vi "Main_22b.vi"() -> ()   [LabVIEW 2023]
uses:
  Cluster_Node.ctl
panel:
  out "Brick Map":map{i32, T1[]}(c390)
  out "Grid":i32[][][](array[numeric])
  out "Array 2":i32[][](array[numeric])
  out "Answer":i32
  in  "Puzzle":string="5,5,156~5,7,156\n8,5,82~8,7,82\n6,5,196~6,7,196\n0,7,7~0,8,7\n2,3,129~2,6,129\n9,5,265~9,7,265\n1,4,278~3,4,278\n2,6,149~4,6,149\n7,7,246~9,7,246\n8,6,282~9,6,282\n1,1,289~1,5,289\n7,3,70~7,6,70\n3,9,278~3,9,280\n6,9,261~7,9,261\n3,5,75~5,5,75\n3,1,221~3,1,224\n0,9,211~2,9,211\n3,9,251~4,9,251\n0,4,28~2,4,28\n2,7,291~2,7,293\n4,3,2~4,5,2\n5,4,96~5,5,96\n5,4,60~5,7,60\n1,2,45~4,2,45\n3,6,145~3,9,145\n9,1,214~9,4,214\n0,4,121~0,6,121\n6,5,22~8,5,22\n2,8,211~4,8,211\n5,0,215~6,0,215\n7,1,80~7,4,80\n4,9,2~6,9,2\n5,8,13~7,8,13\n0,9,210~3,9,210\n6,6,107~6,8,107\n6,7,228~6,9,228\n0,9,96~2,9,96\n0,0,101~0,0,102\n6,4,108~6,6,108\n5,2,237~5,2,240\n1,5,200~1,8,200\n5,9,210~8,9,210\n2,0,28~2,2,28\n2,5,222~4,5,222\n6,7,59~8,7,59\n9,8,152~9,9,152\n0,1,205~0,3,205\n8,7,49~9,7,49\n4,1,44~4,1,47\n0,5,65~0,7,65\n2,2,303~2,3,303\n6,6,21~6,9,21\n4,4,99~4,7,99\n1,0,155~4,0,155\n7,5,15~9,5,15\n4,5,232~4,7,232\n1,9,213~1,9,215\n1,3,105~1,5,105\n4,6,197~4,7,197\n0,6,235~0,7,235\n8,4,303~8,6,303\n3,7,62~5,7,62\n4,2,279~7,2,279\n4,0,45~6,0,45\n8,7,195~8,9,195\n1,7,88~5,7,88\n1,0,246~4,0,246\n5,6,115~5,6,118\n3,3,25~3,5,25\n1,7,261~4,7,261\n7,3,206~8,3,206\n4,1,49~6,1,49\n7,1,179~9,1,179\n6,1,264~8,1,264\n1,8,205~4,8,205\n4,5,283~5,5,283\n3,3,208~3,5,208\n4,1,101~4,1,102\n2,2,272~2,2,274\n4,7,43~4,9,43\n5,7,188~5,9,188\n6,8,290~6,9,290\n3,6,111~6,6,111\n3,4,230~5,4,230\n5,7,154~7,7,154\n8,5,83~9,5,83\n4,2,283~6,2,283\n7,3,276~7,6,276\n6,0,270~8,0,270\n7,7,77~9,7,77\n2,0,256~2,0,258\n3,3,305~3,5,305\n9,7,87~9,9,87\n1,9,219~1,9,221\n3,3,123~3,6,123\n2,2,194~2,2,195\n7,5,64~7,5,67\n1,8,89~1,9,89\n1,0,291~1,2,291\n0,9,166~1,9,166\n2,6,274~2,9,274\n0,6,17~0,6,20\n5,6,277~8,6,277\n4,2,227~4,4,227\n4,6,8~4,7,8\n5,4,84~7,4,84\n1,6,266~1,9,266\n0,7,228~2,7,228\n8,5,29~8,8,29\n1,9,230~2,9,230\n2,1,140~2,3,140\n1,6,3~3,6,3\n2,8,3~2,9,3\n4,0,161~4,2,161\n2,6,254~3,6,254\n5,0,32~5,2,32\n4,0,205~4,2,205\n0,1,161~1,1,161\n2,0,21~5,0,21\n3,1,132~5,1,132\n9,1,10~9,1,10\n7,2,89~7,4,89\n6,0,170~9,0,170\n8,0,145~8,3,145\n1,1,5~3,1,5\n3,5,13~3,7,13\n3,1,30~7,1,30\n7,6,175~7,6,178\n8,4,3~8,5,3\n5,3,113~7,3,113\n2,5,120~3,5,120\n0,0,20~0,3,20\n5,7,47~8,7,47\n3,5,171~3,5,173\n5,4,128~5,7,128\n8,9,211~9,9,211\n3,1,297~5,1,297\n1,9,102~3,9,102\n4,2,47~4,2,47\n4,6,302~4,9,302\n9,3,88~9,3,90\n5,0,26~5,3,26\n7,1,84~8,1,84\n8,1,263~8,3,263\n8,0,95~9,0,95\n2,4,116~2,6,116\n6,4,171~8,4,171\n7,4,245~7,7,245\n4,1,33~6,1,33\n2,2,147~2,4,147\n0,2,276~3,2,276\n5,2,266~8,2,266\n1,3,274~3,3,274\n3,6,193~3,6,196\n0,2,35~3,2,35\n5,4,311~5,5,311\n6,2,274~6,5,274\n9,0,126~9,2,126\n3,4,112~3,6,112\n5,5,163~8,5,163\n6,0,88~8,0,88\n4,0,214~7,0,214\n5,2,35~7,2,35\n4,8,66~7,8,66\n0,8,165~1,8,165\n0,6,180~2,6,180\n4,0,104~6,0,104\n0,5,270~0,8,270\n4,2,73~4,4,73\n3,2,17~5,2,17\n1,5,168~3,5,168\n7,7,22~8,7,22\n6,3,2~6,5,2\n8,3,123~8,5,123\n6,9,142~6,9,143\n7,1,310~9,1,310\n7,1,203~7,4,203\n5,3,272~5,7,272\n1,3,22~1,3,22\n0,9,153~3,9,153\n2,3,285~4,3,285\n1,0,56~1,3,56\n1,8,105~1,9,105\n8,1,128~9,1,128\n1,0,13~1,0,16\n0,6,153~0,8,153\n2,5,95~2,7,95\n6,8,265~8,8,265\n2,1,200~5,1,200\n4,2,307~4,2,309\n1,0,243~3,0,243\n7,1,307~7,4,307\n3,5,99~3,5,102\n3,0,106~4,0,106\n0,1,321~3,1,321\n2,3,199~2,4,199\n6,0,283~6,1,283\n7,2,38~9,2,38\n8,5,16~9,5,16\n0,2,37~0,3,37\n2,2,312~4,2,312\n6,1,225~6,3,225\n1,9,263~1,9,265\n1,6,87~1,8,87\n4,6,40~4,8,40\n4,9,45~7,9,45\n3,1,177~3,1,178\n8,7,14~9,7,14\n4,8,214~7,8,214\n4,7,224~4,9,224\n1,2,245~1,3,245\n8,3,260~8,6,260\n7,7,278~7,8,278\n3,6,212~7,6,212\n0,2,18~0,3,18\n4,6,122~6,6,122\n2,5,12~2,6,12\n7,6,275~7,9,275\n5,5,249~8,5,249\n6,2,83~9,2,83\n4,2,316~6,2,316\n2,6,15~2,6,15\n6,6,248~7,6,248\n7,3,280~9,3,280\n4,8,275~6,8,275\n0,0,77~0,2,77\n6,5,63~8,5,63\n5,0,37~5,0,40\n6,1,75~6,4,75\n4,0,38~4,0,40\n0,8,99~3,8,99\n4,1,298~6,1,298\n7,8,268~9,8,268\n9,1,313~9,3,313\n4,8,24~6,8,24\n5,6,264~5,9,264\n8,3,32~8,5,32\n2,0,205~2,0,207\n0,2,8~2,2,8\n2,7,102~2,7,104\n1,8,239~2,8,239\n8,6,201~9,6,201\n2,1,202~3,1,202\n3,9,62~5,9,62\n8,5,8~8,5,10\n3,9,158~4,9,158\n9,2,143~9,4,143\n8,4,81~8,6,81\n3,9,2~3,9,2\n4,4,67~6,4,67\n3,4,199~3,7,199\n6,8,274~9,8,274\n6,5,58~8,5,58\n9,3,28~9,6,28\n3,1,104~4,1,104\n8,6,23~8,7,23\n2,9,136~4,9,136\n7,0,167~7,3,167\n5,3,11~7,3,11\n6,2,76~6,2,79\n9,0,216~9,2,216\n3,2,255~3,3,255\n0,3,127~0,4,127\n0,1,209~3,1,209\n5,7,191~5,8,191\n5,3,134~5,6,134\n9,2,150~9,2,152\n2,1,295~4,1,295\n1,6,56~1,7,56\n1,9,93~5,9,93\n1,3,24~4,3,24\n5,1,133~7,1,133\n6,8,175~9,8,175\n0,8,272~0,8,274\n0,7,14~0,9,14\n1,7,297~4,7,297\n8,5,68~8,8,68\n2,0,247~5,0,247\n7,2,3~7,2,6\n0,7,247~0,9,247\n4,0,288~6,0,288\n4,6,71~7,6,71\n4,1,57~4,1,59\n2,1,92~4,1,92\n0,4,41~0,6,41\n3,8,287~5,8,287\n3,6,184~5,6,184\n4,3,54~4,4,54\n0,1,208~4,1,208\n0,2,46~1,2,46\n8,4,69~8,5,69\n5,6,113~5,8,113\n6,3,260~6,4,260\n7,3,83~7,4,83\n4,1,170~7,1,170\n0,1,224~0,2,224\n0,4,89~0,6,89\n1,0,9~2,0,9\n6,5,278~6,5,281\n5,2,45~8,2,45\n3,8,155~5,8,155\n2,3,20~4,3,20\n9,2,270~9,4,270\n0,2,127~1,2,127\n1,6,228~3,6,228\n2,3,30~2,5,30\n1,4,124~1,4,126\n1,0,162~1,1,162\n7,2,69~7,3,69\n5,6,198~7,6,198\n2,3,3~2,5,3\n8,1,269~9,1,269\n8,2,146~8,2,147\n0,0,221~3,0,221\n3,8,176~6,8,176\n3,3,83~3,6,83\n7,0,122~8,0,122\n4,4,164~6,4,164\n6,1,106~6,3,106\n3,8,150~5,8,150\n0,6,303~0,7,303\n3,2,205~3,5,205\n4,1,296~4,4,296\n1,8,245~1,9,245\n9,4,156~9,6,156\n6,2,137~6,2,139\n0,3,125~0,5,125\n0,3,29~2,3,29\n0,5,301~3,5,301\n3,9,275~4,9,275\n6,2,173~6,4,173\n8,4,66~8,7,66\n8,8,26~8,9,26\n5,1,90~6,1,90\n2,6,90~4,6,90\n3,4,75~4,4,75\n0,7,239~2,7,239\n6,1,93~6,4,93\n4,4,100~4,4,101\n1,7,67~3,7,67\n4,5,30~4,7,30\n7,2,31~7,4,31\n6,8,221~6,9,221\n6,2,179~8,2,179\n4,7,218~7,7,218\n9,6,277~9,9,277\n2,3,165~2,7,165\n3,4,131~3,4,131\n0,8,243~3,8,243\n0,6,21~0,9,21\n6,0,2~8,0,2\n3,7,101~3,9,101\n4,2,282~5,2,282\n1,5,203~2,5,203\n5,0,172~8,0,172\n7,3,121~7,5,121\n4,0,95~4,2,95\n3,2,313~4,2,313\n8,3,158~8,3,160\n0,5,36~3,5,36\n2,4,80~2,7,80\n0,6,233~0,8,233\n8,0,71~8,2,71\n8,3,307~8,3,307\n4,1,116~4,3,116\n4,2,21~4,2,23\n0,1,227~0,4,227\n1,7,268~1,8,268\n2,6,10~2,8,10\n8,1,131~8,5,131\n3,2,113~5,2,113\n7,7,280~7,9,280\n1,0,130~1,2,130\n3,8,16~5,8,16\n0,3,82~0,4,82\n9,1,315~9,2,315\n4,3,282~6,3,282\n1,5,10~1,7,10\n8,6,97~8,7,97\n0,0,26~0,1,26\n5,0,46~8,0,46\n5,3,36~5,5,36\n7,1,316~7,3,316\n6,6,172~8,6,172\n6,4,56~6,7,56\n2,0,29~3,0,29\n6,1,15~6,3,15\n6,7,102~6,9,102\n0,4,10~2,4,10\n8,2,216~8,3,216\n4,3,70~4,6,70\n0,9,92~1,9,92\n7,1,79~9,1,79\n0,4,285~0,6,285\n2,2,27~2,4,27\n0,2,83~0,4,83\n7,7,228~7,9,228\n9,4,309~9,4,311\n2,0,107~2,1,107\n2,3,293~2,5,293\n7,4,116~8,4,116\n7,4,166~8,4,166\n6,3,78~9,3,78\n3,4,239~5,4,239\n3,2,212~3,4,212\n0,6,147~2,6,147\n0,2,155~0,5,155\n9,4,314~9,7,314\n5,8,137~5,8,138\n8,5,98~8,8,98\n7,7,178~7,8,178\n1,0,58~1,4,58\n7,1,172~7,4,172\n9,6,252~9,6,254\n6,2,287~8,2,287\n0,0,62~2,0,62\n1,5,59~1,7,59\n1,2,249~1,2,250\n1,7,303~1,9,303\n6,3,138~6,3,140\n6,6,113~6,8,113\n6,0,173~7,0,173\n3,4,189~5,4,189\n5,3,247~8,3,247\n6,3,193~6,3,195\n9,2,75~9,2,76\n6,4,140~8,4,140\n4,1,134~4,1,137\n1,6,297~2,6,297\n4,0,165~6,0,165\n0,2,229~0,4,229\n7,5,150~7,7,150\n0,6,230~0,7,230\n2,3,269~5,3,269\n2,7,49~4,7,49\n0,1,216~2,1,216\n8,0,87~8,2,87\n1,0,157~2,0,157\n4,7,130~4,9,130\n5,2,108~5,3,108\n0,6,130~2,6,130\n0,5,33~3,5,33\n2,6,32~5,6,32\n1,6,89~1,6,91\n4,3,275~4,4,275\n3,6,231~6,6,231\n5,3,301~8,3,301\n2,6,173~4,6,173\n2,8,260~4,8,260\n9,3,199~9,6,199\n0,0,255~2,0,255\n3,3,214~3,3,217\n4,7,249~4,9,249\n2,7,271~4,7,271\n1,2,162~1,4,162\n1,4,117~1,7,117\n0,0,219~0,1,219\n4,6,91~7,6,91\n1,1,85~1,4,85\n8,2,128~9,2,128\n7,7,262~9,7,262\n3,3,8~3,3,10\n2,7,242~3,7,242\n8,4,164~8,6,164\n9,2,87~9,2,87\n2,5,256~4,5,256\n7,0,104~9,0,104\n3,8,60~4,8,60\n7,4,115~9,4,115\n1,0,11~1,2,11\n9,7,142~9,7,145\n3,8,17~3,8,20\n2,4,294~4,4,294\n6,5,220~7,5,220\n2,9,22~2,9,25\n4,0,102~7,0,102\n3,7,22~3,7,24\n5,8,199~7,8,199\n0,6,237~0,6,240\n7,6,17~9,6,17\n1,6,196~1,6,198\n8,0,117~8,3,117\n4,4,33~4,4,35\n7,5,307~7,6,307\n5,6,125~5,9,125\n5,2,216~5,2,217\n0,3,294~0,6,294\n4,8,206~7,8,206\n1,3,102~1,5,102\n3,8,63~4,8,63\n9,4,29~9,4,31\n1,0,248~1,2,248\n0,1,282~0,3,282\n2,7,18~2,9,18\n8,4,307~8,6,307\n1,5,40~2,5,40\n5,4,161~5,6,161\n4,8,134~7,8,134\n8,3,64~8,6,64\n0,7,119~0,8,119\n9,6,255~9,6,257\n3,5,98~3,8,98\n6,3,153~8,3,153\n9,0,25~9,3,25\n2,6,296~2,9,296\n4,9,96~5,9,96\n9,1,283~9,4,283\n9,6,120~9,9,120\n4,7,65~5,7,65\n5,9,293~7,9,293\n6,7,151~7,7,151\n4,7,68~6,7,68\n5,2,190~5,5,190\n8,0,80~8,2,80\n4,4,129~6,4,129\n6,3,303~6,6,303\n9,7,219~9,8,219\n4,1,56~5,1,56\n6,3,290~7,3,290\n6,6,101~6,8,101\n8,3,209~8,4,209\n0,8,170~1,8,170\n6,4,13~7,4,13\n2,1,17~2,3,17\n1,6,189~4,6,189\n6,6,209~6,9,209\n8,3,81~9,3,81\n6,2,107~8,2,107\n2,5,286~5,5,286\n6,7,198~6,9,198\n8,6,199~8,7,199\n1,0,3~1,3,3\n3,1,324~5,1,324\n9,5,197~9,6,197\n3,2,79~5,2,79\n9,7,89~9,9,89\n3,8,282~3,9,282\n1,6,176~3,6,176\n7,0,268~9,0,268\n6,3,134~6,6,134\n0,0,252~1,0,252\n5,3,38~8,3,38\n8,0,183~8,1,183\n0,5,16~0,7,16\n3,0,108~4,0,108\n4,9,64~6,9,64\n2,3,143~4,3,143\n0,7,301~2,7,301\n5,9,13~5,9,15\n2,0,78~5,0,78\n2,2,133~4,2,133\n2,9,228~4,9,228\n5,5,34~5,7,34\n5,7,257~5,9,257\n8,3,30~8,5,30\n3,6,96~5,6,96\n3,5,202~6,5,202\n7,0,218~8,0,218\n8,8,88~8,9,88\n5,4,98~7,4,98\n9,0,5~9,2,5\n4,5,87~4,7,87\n0,2,297~0,4,297\n3,7,64~3,8,64\n1,1,234~2,1,234\n6,3,298~6,3,300\n4,7,285~4,9,285\n4,6,227~6,6,227\n4,5,225~4,6,225\n0,2,249~0,4,249\n5,2,107~5,4,107\n6,2,23~9,2,23\n4,8,145~4,9,145\n5,0,285~7,0,285\n1,4,267~1,6,267\n6,3,97~6,5,97\n9,2,173~9,5,173\n6,3,223~6,5,223\n2,0,240~2,2,240\n1,5,259~3,5,259\n5,5,221~5,8,221\n5,4,124~7,4,124\n0,8,187~2,8,187\n7,2,289~7,3,289\n7,3,10~7,4,10\n6,5,175~6,7,175\n7,2,204~7,4,204\n2,4,155~2,4,157\n4,4,209~4,6,209\n4,1,230~4,3,230\n0,6,246~0,9,246\n0,8,16~0,9,16\n4,4,38~4,4,40\n2,6,138~2,9,138\n7,4,174~7,4,176\n5,6,16~8,6,16\n8,1,110~8,1,112\n9,4,141~9,6,141\n3,5,39~3,5,39\n1,4,9~1,7,9\n0,0,122~0,4,122\n5,2,196~5,4,196\n3,3,54~3,3,56\n1,6,226~3,6,226\n9,1,276~9,3,276\n9,7,15~9,9,15\n2,3,295~2,5,295\n8,4,138~8,7,138\n9,2,281~9,3,281\n4,5,292~4,5,293\n2,4,118~2,6,118\n5,0,111~5,2,111\n9,5,63~9,7,63\n4,1,177~6,1,177\n6,2,25~6,3,25\n5,8,56~7,8,56\n9,9,153~9,9,155\n5,1,213~5,3,213\n1,2,301~2,2,301\n5,1,234~5,3,234\n6,1,204~6,2,204\n7,6,45~7,6,45\n6,5,24~6,7,24\n6,2,259~9,2,259\n1,5,154~1,8,154\n4,0,18~4,2,18\n7,6,174~7,9,174\n2,5,82~4,5,82\n9,6,52~9,9,52\n2,9,156~3,9,156\n5,2,72~7,2,72\n3,6,148~3,8,148\n6,1,114~8,1,114\n0,2,167~0,4,167\n1,1,213~1,3,213\n0,1,10~0,3,10\n7,0,215~9,0,215\n7,5,131~7,7,131\n3,0,9~3,1,9\n2,6,57~2,9,57\n4,3,272~4,5,272\n6,0,52~6,0,54\n4,6,246~4,8,246\n1,9,133~4,9,133\n6,4,77~6,4,77\n1,7,230~2,7,230\n9,4,86~9,5,86\n6,8,78~6,9,78\n2,1,206~5,1,206\n5,8,288~8,8,288\n8,5,125~9,5,125\n0,6,175~0,7,175\n6,3,76~9,3,76\n3,3,104~6,3,104\n3,9,11~5,9,11\n1,6,236~1,8,236\n5,4,246~7,4,246\n1,8,168~3,8,168\n0,5,202~0,7,202\n2,0,200~2,0,201\n9,4,216~9,5,216\n9,8,178~9,8,180\n1,2,280~1,5,280\n6,6,153~9,6,153\n1,2,19~1,4,19\n6,6,219~6,8,219\n5,9,77~7,9,77\n0,7,60~0,8,60\n1,6,199~1,8,199\n0,3,158~2,3,158\n2,4,126~4,4,126\n2,4,225~2,7,225\n8,7,284~9,7,284\n3,6,52~3,8,52\n8,1,182~8,1,182\n2,5,264~2,8,264\n6,5,225~6,5,225\n4,6,41~6,6,41\n0,7,162~3,7,162\n0,4,196~0,6,196\n5,9,83~8,9,83\n3,7,11~5,7,11\n0,7,13~2,7,13\n5,0,160~5,0,162\n1,4,277~3,4,277\n7,1,104~7,1,107\n6,3,269~6,4,269\n5,6,5~5,8,5\n3,9,8~6,9,8\n3,0,1~3,2,1\n1,7,175~3,7,175\n3,3,151~6,3,151\n7,1,158~9,1,158\n6,3,12~7,3,12\n0,1,164~0,2,164\n9,4,175~9,5,175\n3,9,64~3,9,66\n1,8,172~3,8,172\n3,5,41~3,5,41\n8,4,292~8,4,295\n0,6,74~0,8,74\n9,3,83~9,4,83\n4,4,31~4,5,31\n6,0,264~8,0,264\n4,3,21~5,3,21\n3,8,10~5,8,10\n3,9,283~5,9,283\n2,3,304~4,3,304\n0,3,208~0,3,210\n6,4,111~6,4,113\n3,3,75~5,3,75\n3,9,272~5,9,272\n2,6,248~4,6,248\n3,9,265~5,9,265\n9,0,26~9,0,27\n9,3,306~9,5,306\n8,5,281~8,7,281\n7,1,277~7,3,277\n3,4,195~4,4,195\n7,8,30~9,8,30\n9,5,202~9,6,202\n3,8,55~3,8,57\n6,0,51~6,1,51\n0,4,132~1,4,132\n7,0,13~9,0,13\n0,4,118~0,7,118\n8,7,123~8,7,126\n0,1,124~0,1,126\n3,2,57~6,2,57\n5,0,269~7,0,269\n5,5,280~5,7,280\n2,7,82~4,7,82\n4,0,133~4,1,133\n1,9,165~1,9,165\n1,6,125~3,6,125\n4,9,139~7,9,139\n1,2,14~1,3,14\n5,7,251~8,7,251\n4,7,12~4,7,14\n5,5,261~5,8,261\n6,0,5~8,0,5\n4,2,134~6,2,134\n6,1,280~8,1,280\n2,9,21~2,9,21\n0,0,293~2,0,293\n7,9,86~9,9,86\n3,3,240~3,5,240\n7,4,113~7,7,113\n4,3,7~4,5,7\n0,0,223~0,2,223\n8,8,69~8,8,72\n0,7,8~0,7,10\n2,0,35~5,0,35\n6,6,123~6,8,123\n4,7,134~7,7,134\n6,7,110~7,7,110\n3,6,158~5,6,158\n6,6,20~6,9,20\n6,3,284~6,5,284\n8,2,134~8,3,134\n0,6,287~0,6,287\n1,7,14~1,8,14\n0,6,181~0,8,181\n0,7,18~0,8,18\n7,0,118~9,0,118\n7,9,80~9,9,80\n6,1,2~9,1,2\n0,6,195~2,6,195\n3,7,84~5,7,84\n5,2,207~5,3,207\n7,5,201~7,6,201\n2,1,56~2,3,56\n6,2,212~9,2,212\n6,2,33~6,4,33\n4,5,270~7,5,270\n0,3,49~3,3,49\n4,3,273~4,5,273\n1,7,164~1,9,164\n0,1,253~0,2,253\n8,4,83~8,4,85\n8,5,120~8,7,120\n6,1,35~8,1,35\n5,3,152~5,3,155\n2,3,84~2,5,84\n2,7,208~2,9,208\n5,1,173~9,1,173\n2,2,285~4,2,285\n6,6,130~8,6,130\n8,3,140~8,3,142\n1,3,2~1,5,2\n5,0,211~5,3,211\n1,1,167~3,1,167\n7,1,75~7,3,75\n4,0,43~4,2,43\n0,6,146~3,6,146\n8,1,189~8,1,191\n0,8,4~0,9,4\n2,2,157~2,3,157\n2,7,278~2,7,279\n1,1,131~3,1,131\n1,4,210~1,6,210\n3,1,318~4,1,318\n9,7,227~9,9,227\n1,3,121~1,5,121\n3,1,107~3,2,107\n3,9,192~3,9,194\n7,7,147~9,7,147\n1,1,164~1,2,164\n1,1,86~3,1,86\n4,0,270~5,0,270\n8,0,125~9,0,125\n0,3,177~0,7,177\n3,2,209~5,2,209\n2,3,290~2,4,290\n5,2,165~5,4,165\n5,5,187~5,7,187\n0,1,217~0,2,217\n2,5,169~2,5,169\n0,4,2~0,6,2\n9,6,149~9,8,149\n7,5,5~7,7,5\n5,6,123~5,8,123\n8,2,210~8,4,210\n9,4,268~9,6,268\n1,3,211~1,5,211\n2,9,287~4,9,287\n5,3,279~7,3,279\n2,1,118~4,1,118\n5,2,208~6,2,208\n6,0,1~9,0,1\n6,3,245~6,4,245\n0,5,266~2,5,266\n1,2,120~1,5,120\n0,1,168~0,2,168\n6,3,7~8,3,7\n6,3,213~8,3,213\n1,2,131~2,2,131\n6,5,95~6,7,95\n3,4,279~3,6,279\n0,4,115~2,4,115\n1,1,62~1,3,62\n2,7,168~4,7,168\n8,7,254~8,9,254\n7,7,160~9,7,160\n7,7,177~9,7,177\n2,6,197~2,7,197\n3,9,191~5,9,191\n3,2,20~6,2,20\n0,3,204~2,3,204\n0,9,298~3,9,298\n2,1,299~4,1,299\n4,0,158~6,0,158\n2,2,136~2,2,137\n3,6,91~3,9,91\n6,6,143~9,6,143\n4,3,191~6,3,191\n1,8,210~3,8,210\n3,7,85~5,7,85\n9,4,21~9,4,24\n5,5,21~5,7,21\n5,5,191~5,6,191\n4,5,76~4,7,76\n7,2,314~9,2,314\n1,5,80~1,6,80\n4,6,104~7,6,104\n3,3,186~3,6,186\n3,3,291~5,3,291\n0,2,281~0,3,281\n6,1,318~8,1,318\n5,1,233~5,4,233\n7,5,20~7,7,20\n3,3,84~3,5,84\n3,2,12~5,2,12\n0,4,172~2,4,172\n8,7,278~8,8,278\n7,9,310~9,9,310\n1,1,237~3,1,237\n6,3,266~8,3,266\n4,9,4~4,9,6\n2,5,242~6,5,242\n1,8,20~1,8,22\n6,6,249~9,6,249\n1,2,205~1,5,205\n1,0,244~3,0,244\n2,2,304~5,2,304\n3,0,8~5,0,8\n6,3,304~9,3,304\n0,6,283~2,6,283\n6,3,83~6,5,83\n3,8,153~3,8,153\n3,8,54~6,8,54\n4,4,317~7,4,317\n2,5,265~2,5,265\n9,2,272~9,4,272\n2,5,98~2,7,98\n0,3,201~0,6,201\n1,5,201~1,7,201\n7,7,76~9,7,76\n0,1,278~0,2,278\n6,6,98~6,7,98\n3,4,236~6,4,236\n1,1,219~3,1,219\n6,3,87~6,5,87\n3,8,271~4,8,271\n4,3,251~4,6,251\n9,6,50~9,7,50\n1,7,275~4,7,275\n1,7,118~1,7,120\n2,6,172~3,6,172\n1,6,157~1,8,157\n6,3,164~9,3,164\n4,4,258~7,4,258\n2,1,192~2,4,192\n6,0,77~6,1,77\n0,0,171~0,1,171\n9,5,270~9,5,273\n0,5,204~0,5,207\n8,6,262~8,6,265\n9,3,177~9,4,177\n0,8,182~2,8,182\n7,1,315~7,4,315\n8,5,95~8,6,95\n8,6,196~8,7,196\n2,7,87~2,9,87\n7,2,109~9,2,109\n7,3,156~7,5,156\n7,1,176~7,3,176\n8,1,90~8,2,90\n7,2,263~7,2,263\n4,3,221~4,5,221\n5,1,116~7,1,116\n9,6,65~9,9,65\n2,3,111~5,3,111\n9,2,146~9,5,146\n0,1,251~0,3,251\n5,4,57~6,4,57\n0,4,190~3,4,190\n2,8,288~4,8,288\n1,1,99~1,3,99\n8,6,151~8,8,151\n3,6,269~3,9,269\n5,3,205~5,5,205\n4,0,203~4,1,203\n8,2,289~8,4,289\n1,6,16~1,8,16\n5,4,244~5,6,244\n0,6,151~0,7,151\n4,4,64~6,4,64\n5,0,11~7,0,11\n8,2,250~8,3,250\n2,3,281~2,6,281\n4,0,10~6,0,10\n0,0,79~0,2,79\n1,1,269~3,1,269\n7,5,60~9,5,60\n2,3,272~2,3,273\n4,1,224~4,4,224\n8,2,79~8,3,79\n7,6,116~7,8,116\n1,3,288~4,3,288\n9,2,10~9,4,10\n0,3,40~0,5,40\n5,3,294~7,3,294\n5,3,67~8,3,67\n0,8,206~0,9,206\n9,2,274~9,4,274\n6,6,305~6,6,307\n6,6,140~6,8,140\n2,3,276~2,5,276\n2,3,297~3,3,297\n6,5,110~6,5,112\n9,3,200~9,3,202\n5,5,132~7,5,132\n7,4,11~9,4,11\n8,8,31~8,8,33\n2,4,226~2,5,226\n9,2,79~9,2,82\n6,6,42~7,6,42\n6,8,216~9,8,216\n5,6,256~5,8,256\n4,5,228~4,5,229\n9,5,196~9,7,196\n0,9,22~0,9,22\n7,6,74~7,9,74\n5,3,273~7,3,273\n8,5,13~8,8,13\n7,0,81~7,2,81\n5,8,231~6,8,231\n0,4,208~0,4,208\n5,1,282~7,1,282\n7,2,100~7,4,100\n4,1,23~7,1,23\n0,0,100~2,0,100\n4,5,132~4,8,132\n2,7,136~5,7,136\n4,5,218~6,5,218\n8,8,221~9,8,221\n6,8,262~6,8,264\n3,5,147~3,7,147\n5,9,5~5,9,6\n8,2,162~8,5,162\n2,7,170~2,7,173\n4,3,114~5,3,114\n4,0,135~7,0,135\n5,3,14~8,3,14\n5,4,62~5,6,62\n2,2,102~4,2,102\n0,3,248~0,6,248\n1,8,270~1,9,270\n1,2,278~1,3,278\n3,6,127~3,7,127\n9,1,7~9,3,7\n1,3,35~4,3,35\n0,1,294~0,1,295\n5,5,94~5,8,94\n5,7,193~9,7,193\n6,8,25~8,8,25\n7,8,258~7,9,258\n6,1,32~6,4,32\n8,6,257~8,7,257\n2,0,58~5,0,58\n5,0,77~5,2,77\n0,3,85~0,4,85\n0,5,153~2,5,153\n9,2,262~9,2,263\n2,1,296~2,1,298\n2,0,102~2,0,105\n3,8,291~3,8,291\n7,2,118~7,4,118\n4,6,18~7,6,18\n5,5,8~5,7,8\n1,5,233~1,7,233\n6,0,101~6,2,101\n9,5,158~9,7,158\n0,2,287~0,4,287\n3,5,302~5,5,302\n0,2,1~0,5,1\n1,1,294~1,3,294\n3,1,176~5,1,176\n3,5,266~3,8,266\n5,4,309~7,4,309\n5,2,175~7,2,175\n3,4,172~5,4,172\n4,3,100~6,3,100\n5,6,57~5,7,57\n2,1,273~4,1,273\n2,3,146~4,3,146\n6,6,118~9,6,118\n2,6,183~4,6,183\n4,1,201~4,3,201\n8,0,186~8,2,186\n4,6,259~4,9,259\n1,4,133~1,4,134\n3,1,113~5,1,113\n3,6,252~5,6,252\n4,3,306~4,5,306\n8,7,179~9,7,179\n0,4,199~0,5,199\n3,4,127~4,4,127\n3,3,262~3,5,262\n0,1,81~0,4,81\n0,2,125~0,2,126\n2,3,317~2,5,317\n4,3,118~6,3,118\n1,7,238~3,7,238\n1,3,32~3,3,32\n0,6,68~0,7,68\n7,4,297~8,4,297\n8,6,175~8,7,175\n1,4,169~1,7,169\n1,3,216~1,3,218\n1,6,263~1,6,265\n8,4,70~8,4,73\n2,2,74~4,2,74\n5,4,277~6,4,277\n4,0,234~4,2,234\n0,6,55~2,6,55\n8,2,167~8,2,169\n5,2,166~8,2,166\n5,6,253~7,6,253\n0,6,204~0,6,204\n2,3,154~2,5,154\n2,7,83~2,9,83\n2,7,6~4,7,6\n0,8,203~2,8,203\n2,1,58~2,2,58\n3,9,142~5,9,142\n9,2,2~9,3,2\n4,2,156~4,3,156\n5,8,68~6,8,68\n1,5,78~3,5,78\n6,6,304~7,6,304\n6,8,259~7,8,259\n5,7,194~5,7,196\n0,1,193~0,2,193\n8,7,99~8,7,101\n5,8,3~5,8,3\n8,0,92~8,3,92\n5,5,137~5,5,140\n4,1,284~5,1,284\n6,3,73~7,3,73\n4,9,92~6,9,92\n5,6,293~5,7,293\n9,3,140~9,7,140\n5,8,6~5,8,8\n6,1,122~6,2,122\n9,8,134~9,9,134\n4,9,78~5,9,78\n9,1,148~9,3,148\n7,9,3~8,9,3\n0,7,3~0,8,3\n2,2,11~4,2,11\n0,1,53~2,1,53\n1,7,121~4,7,121\n7,9,5~8,9,5\n2,0,61~2,1,61\n9,8,222~9,8,224\n6,4,88~7,4,88\n4,9,128~8,9,128\n6,5,248~8,5,248\n4,2,58~5,2,58\n6,0,121~8,0,121\n0,9,218~3,9,218\n6,1,180~6,1,180\n3,5,267~3,7,267\n5,2,284~6,2,284\n3,6,55~6,6,55\n0,3,71~0,6,71\n7,8,180~7,9,180\n5,9,67~5,9,68\n7,3,283~7,5,283\n3,2,300~3,4,300\n8,0,288~8,2,288\n3,3,254~6,3,254\n5,2,74~5,5,74\n0,7,184~0,9,184\n2,1,270~2,1,270\n6,7,276~8,7,276\n2,1,51~4,1,51\n3,5,227~3,8,227\n2,8,158~5,8,158\n5,7,119~7,7,119\n1,6,19~1,8,19\n9,7,226~9,8,226\n6,0,256~6,3,256\n4,6,262~4,6,262\n7,6,159~9,6,159\n4,4,114~4,7,114\n0,2,191~0,4,191\n5,7,248~8,7,248\n4,9,277~7,9,277\n5,5,227~7,5,227\n3,5,28~4,5,28\n1,2,97~5,2,97\n8,2,43~8,2,43\n6,6,94~6,8,94\n2,5,298~2,5,300\n2,9,221~4,9,221\n7,4,225~7,7,225\n1,1,51~1,3,51\n3,7,37~5,7,37\n7,1,71~7,4,71\n2,0,152~3,0,152\n1,2,281~1,5,281\n8,1,156~8,4,156\n3,1,98~6,1,98\n0,0,57~3,0,57\n7,1,25~7,3,25\n5,6,223~7,6,223\n4,3,101~6,3,101\n4,2,281~6,2,281\n7,1,109~8,1,109\n2,3,229~2,5,229\n5,6,126~5,7,126\n4,5,245~4,6,245\n1,5,149~1,6,149\n5,9,70~7,9,70\n1,2,219~1,4,219\n0,4,168~0,7,168\n1,4,82~3,4,82\n2,6,166~2,7,166\n6,3,297~6,5,297\n4,8,81~4,9,81\n5,9,175~8,9,175\n5,7,3~6,7,3\n0,2,159~0,4,159\n1,9,261~4,9,261\n6,6,126~6,6,128\n6,1,28~6,4,28\n3,0,167~5,0,167\n2,0,2~4,0,2\n6,9,255~9,9,255\n9,0,29~9,0,29\n0,0,174~0,0,176\n3,2,99~5,2,99\n0,7,170~0,7,172\n9,3,91~9,3,94\n4,6,121~6,6,121\n5,4,242~7,4,242\n4,4,193~6,4,193\n2,0,203~2,0,203\n0,4,49~2,4,49\n6,7,279~7,7,279\n4,0,90~4,2,90\n9,6,121~9,7,121\n4,4,257~4,7,257\n1,0,97~4,0,97\n3,2,213~3,2,217\n3,3,4~6,3,4\n0,6,57~0,7,57\n2,0,10~2,0,11\n7,8,75~7,8,78\n8,2,180~8,4,180\n4,5,117~7,5,117\n4,3,57~4,3,58\n2,6,92~2,6,94\n0,4,113~3,4,113\n8,2,174~8,5,174\n8,2,40~8,4,40\n4,1,55~4,3,55\n5,8,271~7,8,271\n7,4,170~9,4,170\n7,6,94~9,6,94\n8,4,213~8,5,213\n2,7,19~3,7,19\n1,2,5~1,5,5\n0,4,268~0,7,268\n5,5,275~7,5,275\n8,4,299~8,6,299\n7,2,70~9,2,70\n8,6,306~8,9,306\n0,4,296~0,6,296\n1,4,262~1,6,262\n8,4,300~8,6,300\n8,4,155~8,6,155\n4,5,115~7,5,115\n7,0,261~7,2,261\n1,5,302~2,5,302\n2,0,198~2,2,198\n9,5,21~9,7,21\n6,2,1~6,2,3\n3,2,153~6,2,153\n2,2,269~4,2,269\n0,5,295~0,6,295\n1,1,47~1,4,47\n0,0,256~0,0,259\n0,7,86~3,7,86\n4,5,124~7,5,124\n1,4,128~1,4,130\n3,7,305~5,7,305\n0,7,295~2,7,295\n6,9,89~7,9,89\n3,0,149~3,4,149\n9,3,203~9,5,203\n0,5,62~0,8,62\n8,5,6~8,7,6\n6,8,136~6,8,139\n6,3,137~9,3,137\n3,3,86~3,4,86\n3,6,241~3,8,241\n1,7,7~4,7,7\n2,2,315~2,5,315\n3,3,298~3,5,298\n7,6,3~7,7,3\n0,1,22~0,1,23\n8,8,309~8,9,309\n1,1,150~3,1,150\n6,7,222~8,7,222\n3,1,115~3,2,115\n0,1,60~1,1,60\n6,7,260~8,7,260\n0,6,291~2,6,291\n0,4,204~2,4,204\n2,3,38~4,3,38\n7,7,148~9,7,148\n2,7,300~4,7,300\n0,5,203~0,7,203\n1,2,16~1,2,17\n4,6,207~4,9,207\n1,7,161~4,7,161\n5,4,274~5,6,274\n8,2,93~8,4,93\n3,3,128~3,5,128\n1,0,6~3,0,6\n3,6,61~3,9,61\n5,1,201~7,1,201\n3,0,170~3,1,170\n3,1,268~3,4,268\n1,4,292~1,6,292\n4,7,46~6,7,46\n1,0,158~1,2,158\n2,2,196~2,3,196\n5,4,260~5,5,260\n5,1,4~7,1,4\n6,3,198~6,4,198\n7,5,177~9,5,177\n3,6,290~5,6,290\n6,0,217~6,0,219\n7,2,213~7,2,213\n6,6,136~8,6,136\n5,5,267~5,8,267\n8,6,9~8,7,9\n2,7,141~2,9,141\n2,2,299~4,2,299\n1,4,7~1,6,7\n8,9,131~9,9,131\n0,7,244~0,9,244\n9,0,72~9,3,72\n3,9,273~5,9,273\n8,0,116~8,2,116\n9,3,19~9,5,19\n5,5,78~8,5,78\n0,0,251~2,0,251\n7,1,205~9,1,205\n3,3,23~3,6,23\n6,8,14~8,8,14\n4,5,195~4,7,195\n0,9,299~2,9,299\n8,2,137~8,2,139\n0,0,74~0,2,74\n5,9,47~8,9,47\n3,2,265~3,5,265\n2,0,210~4,0,210\n3,6,129~3,8,129\n4,4,289~4,6,289\n6,3,215~8,3,215\n0,2,15~4,2,15\n3,4,263~3,6,263\n5,5,215~5,7,215\n3,4,170~3,6,170\n2,3,51~5,3,51\n1,4,37~1,7,37\n2,2,33~5,2,33\n2,1,87~5,1,87\n0,5,251~0,6,251\n0,5,150~0,9,150\n5,3,3~8,3,3\n1,6,207~1,9,207\n1,7,100~4,7,100\n2,6,53~5,6,53\n7,1,13~7,1,15\n6,6,308~6,7,308\n3,4,103~5,4,103\n5,4,4~5,7,4\n6,5,82~6,6,82\n8,1,124~8,4,124\n4,6,79~6,6,79\n4,0,20~4,1,20\n8,4,169~8,7,169\n9,2,85~9,3,85\n8,6,166~8,8,166\n0,2,243~2,2,243\n6,8,260~8,8,260\n4,9,226~6,9,226\n1,2,150~4,2,150\n4,4,79~7,4,79\n8,3,120~8,4,120\n3,0,94~3,1,94\n7,5,315~9,5,315\n8,2,118~8,2,120\n3,4,104~4,4,104\n1,1,232~4,1,232\n7,1,77~7,2,77\n1,4,159~1,7,159\n8,4,25~8,6,25\n4,9,97~4,9,99\n2,6,192~4,6,192\n6,1,118~6,1,119\n4,5,253~4,5,255\n9,0,266~9,3,266\n2,1,153~2,1,154\n2,7,3~4,7,3\n8,1,291~8,2,291\n0,2,206~0,4,206\n0,2,73~0,3,73\n2,7,15~2,9,15\n7,2,28~7,4,28\n6,1,10~8,1,10\n0,1,293~3,1,293\n1,1,20~2,1,20\n2,4,289~2,7,289\n4,1,317~7,1,317\n0,6,87~0,9,87\n6,1,7~6,1,7\n7,6,254~7,7,254\n3,3,6~3,3,6\n7,1,102~7,3,102\n4,3,147~6,3,147\n7,0,137~7,0,141\n1,2,27~1,4,27\n6,9,49~8,9,49\n5,0,2~5,0,3\n1,6,172~1,6,175\n0,5,302~0,5,305"
  in  "Example":string="1,0,1~1,2,1\n0,0,2~2,0,2\n0,2,3~2,2,3\n0,0,4~0,2,4\n2,0,5~2,2,5\n0,1,6~2,1,6\n1,1,8~1,1,9"
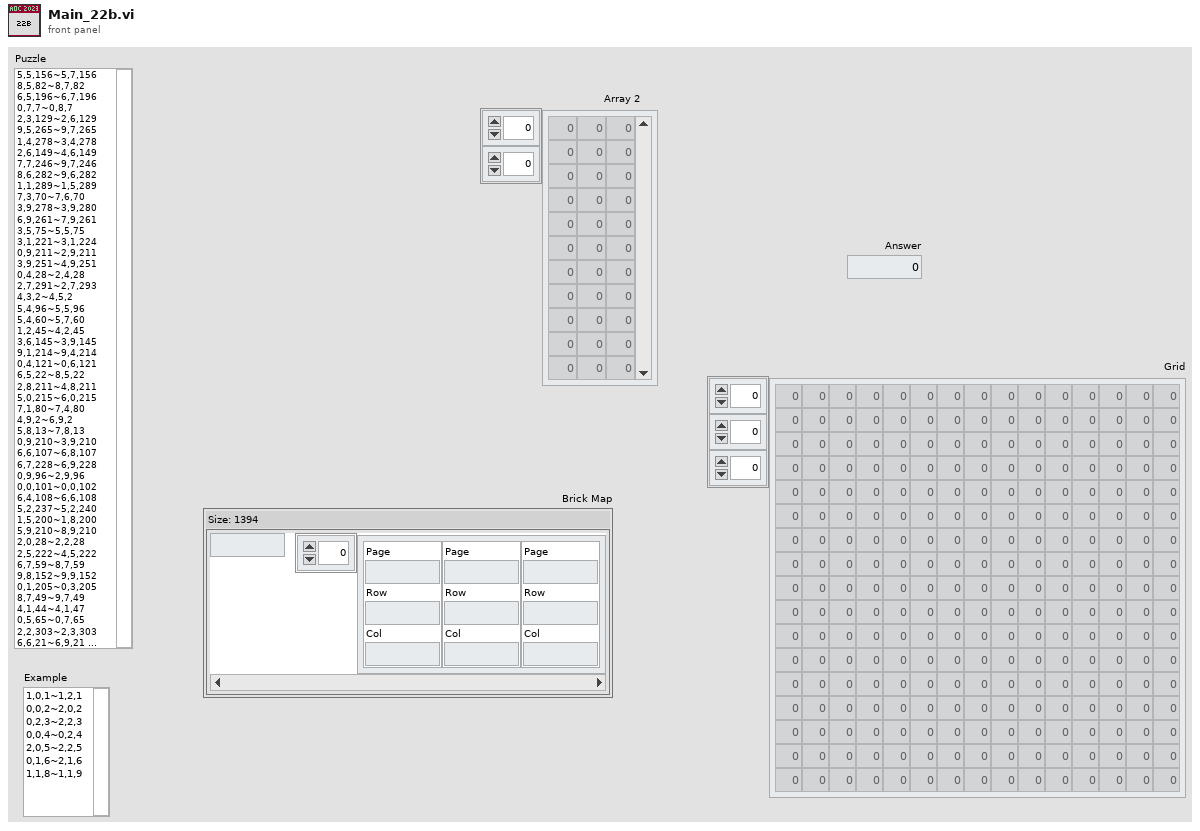
[diagram p1: front panel]
types:
  T1 = typedef "Cluster_Node.ctl" = cluster{"Page":i32, "Row":i32, "Col":i32}
  T2 = typedef "Cluster_Dependencies.ctl" = cluster{"keep":bool, "Dependancies":i32[]}
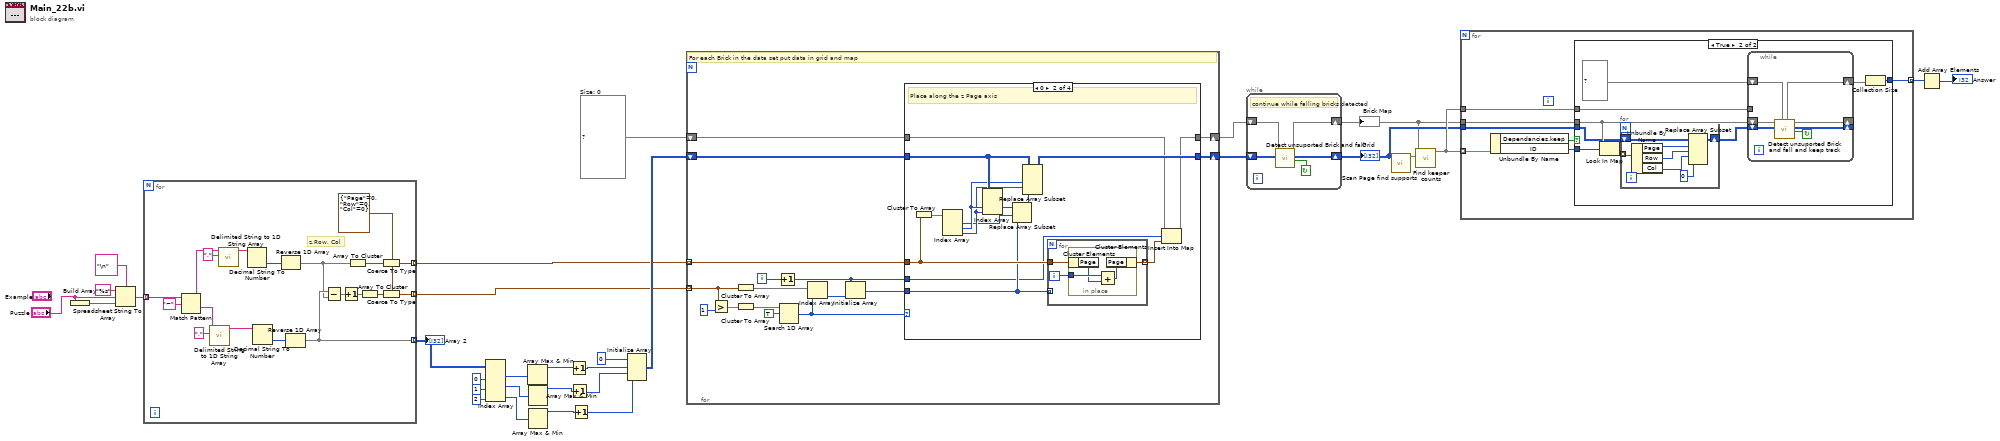
[diagram p0: block diagram]
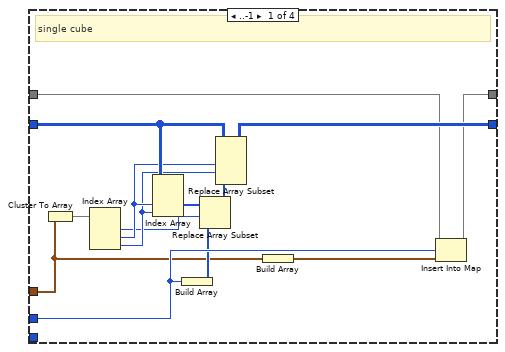
[diagram p2: hidden frame]
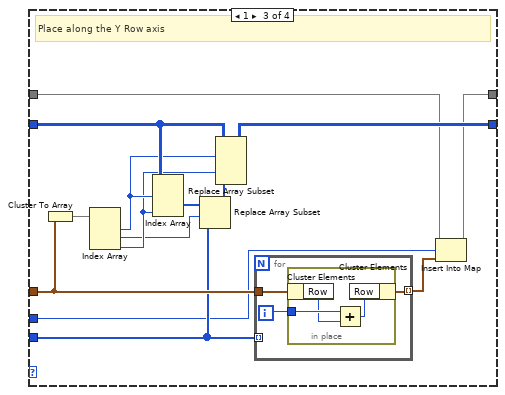
[diagram p3: hidden frame]
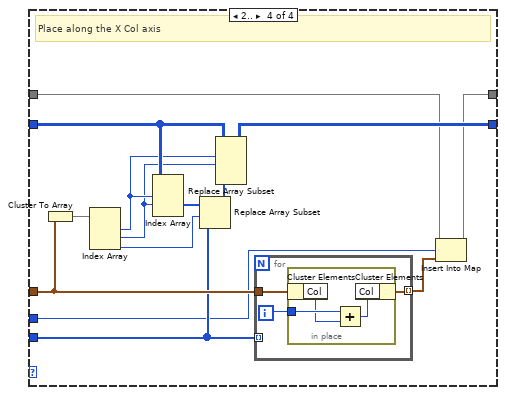
[diagram p4: hidden frame]
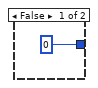
[diagram p5: hidden frame]
diagram:
  w10 = map{i32, T1[]} {}  # Size: 0
  n1 = Build Array("Puzzle") -> (w31:string[])
  n2 = Spreadsheet String To Array(delimiter (Tab)="\n", format string="%s", spreadsheet string="Puzzle", array type (2D Dbl)=w31) -> (array=w28:string[])
  n3 = for {
    tunnel: w28 -> [w50] mode=indexing
    tunnel: [w36] -> w12 mode=indexing
    tunnel: [w39] -> w27 mode=indexing
    tunnel: [w33] -> w11 mode=indexing
    w32 = T1 {"Page"=0, "Row"=0, "Col"=0} ("Point")
    # "z,Row, Col"
    n4 = Match Pattern(string=w50, regular expression="~") -> (before substring=w48:string, after substring=w46:string)  [unwired: 1 in, 2 out]
    n5 = call <vilib>:"Delimited String to 1D String Array.vi"("delimiter"=",", "delimited string"=w46) -> ("string array"=w43:string[])  [unwired: 9 in]
    n6 = call <vilib>:"Delimited String to 1D String Array.vi"("delimiter"=",", "delimited string"=w48) -> ("string array"=w44:string[])  [unwired: 9 in]
    n7 = Decimal String To Number(string=w44) -> (number=w41:i32[])  [unwired: 2 in, 1 out]
    n8 = Decimal String To Number(string=w43) -> (number=w40:i32[])  [unwired: 2 in, 1 out]
    n9 = Reverse 1D Array(array=w41) -> (reversed array=w37:i32[])
    n10 = Reverse 1D Array(array=w40) -> (reversed array=w39:i32[])
    n11 = Subtract(x=w39, y=w37) -> (x-y=w42:i32[])
    n12 = Increment(x=w42) -> (x+1=w34:i32[])
    n13 = Array To Cluster(array=w37) -> (cluster=w38:cluster{"[0]":i32, "[1]":i32, "[2]":i32})
    n14 = Array To Cluster(array=w34) -> (cluster=w35:cluster{"[0]":i32, "[1]":i32, "[2]":i32})
    n15 = Coerce To Type(0:w38, 1:w32) -> (2:w36:T1)
    n16 = Coerce To Type(0:w35, 1:w32) -> (2:w33:T1)
  }
  "Array 2" <- w27
  n17 = Index Array(array=w27, index (col) #1=0 ("disabled index (col)"), index (col) #2=1 ("index (col)"), index (col) #3=2 ("index (col)")) -> (element #1=w21:i32[], element #2=w22:i32[], element #3=w23:i32[])  [unwired: 3 in]
  n18 = Array Max & Min(array=w21) -> (max value=w20:i32)  [unwired: 3 out]
  n19 = Array Max & Min(array=w22) -> (max value=w19:i32)  [unwired: 3 out]
  n20 = Array Max & Min(array=w23) -> (max value=w18:i32)  [unwired: 3 out]
  n21 = Increment(x=w20) -> (x+1=w17:i32)
  n22 = Increment(x=w19) -> (x+1=w16:i32)
  n23 = Increment(x=w18) -> (x+1=w15:i32)
  n24 = Initialize Array(0 ("max value"), w17, w16, w15) -> (w13:i32[][][])
  n25 = for {
    shift-right: [w58] -> w9
    shift-left: w13 -> [w60]
    tunnel: w12 -> [w59] mode=indexing
    tunnel: w11 -> [w54] mode=indexing
    shift-right: [w51] -> w8
    shift-left: w10 -> [w52]
    i -> [w62]
    # "For each Brick in the data set put data in grid and map"
    n26 = Greater?(x=w54, y=1 ("String")) -> (0:w56:cluster{"Page":bool, "Row":bool, "Col":bool})
    n27 = Cluster To Array(cluster=w54) -> (array=w55:i32[])
    n28 = Cluster To Array(cluster=w56) -> (array=w57:bool[])
    n29 = Increment(x=w62) -> (x+1=w53:i32)
    n30 = Search 1D Array(1D array=w57, element=TRUE) -> (index of element=w64:i32)  [unwired: 1 in]
    n31 = Index Array(array=w55, index=w64) -> (element=w63:i32)
    n32 = Initialize Array(w53, w63) -> (w61:i32[])
    n33 = case shown="0" w64 {
      tunnel: w61 -> [_ w87 w107 w125]
      tunnel: w60 -> [w80 w94 w114 w134]
      tunnel: w59 -> [w68 w88 w108 w126]
      tunnel: [w77 w91 w111 w131] -> w58
      tunnel: w53 -> [w70 w84 w104 w122]
      tunnel: w52 -> [w74 w86 w106 w124]
      tunnel: [w73 w85 w105 w123] -> w51
      frame ..-1 {
        # "single cube"
        n34 = Cluster To Array(cluster=w68) -> (array=w75:i32[])
        n35 = Index Array(array=w75) -> (element #1=w71:i32, element #2=w76:i32, element #3=w72:i32)  [unwired: 3 in]
        n36 = Index Array(array=w80, index (dim 1)=w76, index (dim 2)=w72) -> (element=w79:i32[])  [unwired: 1 in]
        n37 = Build Array(w70) -> (w69:i32[])
        n38 = Replace Array Subset(array=w79, new element=w69, index=w71) -> (w78:i32[])
        n39 = Replace Array Subset(array=w80, new element=w78, index (dim 1)=w76, index (dim 2)=w72) -> (w77:i32[][][])  [unwired: 1 in]
        n40 = Build Array(w68) -> (w67:T1[])
        n41 = Insert Into Map(map in=w74, key=w70, value=w67) -> (map out=w73:map{i32, T1[]})  [unwired: 2 out]
      }
      frame 0 {
        # "Place along the z Page axis"
        n42 = Cluster To Array(cluster=w88) -> (array=w89:i32[])
        n43 = Index Array(array=w89) -> (element #1=w81:i32, element #2=w90:i32, element #3=w82:i32)  [unwired: 3 in]
        n44 = Index Array(array=w94, index (dim 1)=w90, index (dim 2)=w82) -> (element=w93:i32[])  [unwired: 1 in]
        n45 = Replace Array Subset(array=w93, new element=w87, index=w81) -> (w92:i32[])
        n46 = Replace Array Subset(array=w94, new element=w92, index (dim 1)=w90, index (dim 2)=w82) -> (w91:i32[][][])  [unwired: 1 in]
        n47 = for {
          tunnel: w88 -> [w96]
          tunnel: [w95] -> w83 mode=indexing
          tunnel: w87 -> [_] mode=indexing
          i -> [w97]
          n48 = in-place {
            in-place-border: w97 -> [w100]
            n49 = in-place-cluster #1(w96) -> ("Page"=w99:i32)
            n50 = Add(x=w100, y=w99) -> (x+y=w98:i32)
            n51 = in-place-cluster #1("Page"=w98) -> (w95:T1)
          }
        }
        n52 = Insert Into Map(map in=w86, key=w84, value=w83) -> (map out=w85:map{i32, T1[]})  [unwired: 2 out]
      }
      frame 1 {
        # "Place along the Y Row axis"
        n53 = Cluster To Array(cluster=w108) -> (array=w109:i32[])
        n54 = Index Array(array=w109) -> (element #1=w110:i32, element #2=w101:i32, element #3=w102:i32)  [unwired: 3 in]
        n55 = Index Array(array=w114, index (dim 0)=w110, index (dim 2)=w102) -> (element=w113:i32[])  [unwired: 1 in]
        n56 = Replace Array Subset(array=w113, new element=w107, index=w101) -> (w112:i32[])
        n57 = Replace Array Subset(array=w114, new element=w112, index (dim 0)=w110, index (dim 2)=w102) -> (w111:i32[][][])  [unwired: 1 in]
        n58 = for {
          tunnel: w108 -> [w116]
          tunnel: [w115] -> w103 mode=indexing
          tunnel: w107 -> [_] mode=indexing
          i -> [w117]
          n59 = in-place {
            in-place-border: w117 -> [w120]
            n60 = in-place-cluster #2(w116) -> ("Row"=w119:i32)
            n61 = Add(x=w120, y=w119) -> (x+y=w118:i32)
            n62 = in-place-cluster #2("Row"=w118) -> (w115:T1)
          }
        }
        n63 = Insert Into Map(map in=w106, key=w104, value=w103) -> (map out=w105:map{i32, T1[]})  [unwired: 2 out]
      }
      frame 2.. {
        # "Place along the X Col axis"
        n64 = Cluster To Array(cluster=w126) -> (array=w127:i32[])
        n65 = Index Array(array=w127) -> (element #1=w129:i32, element #2=w128:i32, element #3=w130:i32)  [unwired: 3 in]
        n66 = Index Array(array=w134, index (dim 0)=w129, index (dim 1)=w128) -> (element=w133:i32[])  [unwired: 1 in]
        n67 = Replace Array Subset(array=w133, new element=w125, index=w130) -> (w132:i32[])
        n68 = Replace Array Subset(array=w134, new element=w132, index (dim 0)=w129, index (dim 1)=w128) -> (w131:i32[][][])  [unwired: 1 in]
        n69 = for {
          tunnel: w126 -> [w136]
          tunnel: [w135] -> w121 mode=indexing
          tunnel: w125 -> [_] mode=indexing
          i -> [w137]
          n70 = in-place {
            in-place-border: w137 -> [w140]
            n71 = in-place-cluster #3(w136) -> ("Col"=w139:i32)
            n72 = Add(x=w140, y=w139) -> (x+y=w138:i32)
            n73 = in-place-cluster #3("Col"=w138) -> (w135:T1)
          }
        }
        n74 = Insert Into Map(map in=w124, key=w122, value=w121) -> (map out=w123:map{i32, T1[]})  [unwired: 2 out]
      }
    }
  }
  n75 = while {
    shift-right: [w144] -> w2
    shift-left: w8 -> [w145]
    shift-right: [w143] -> w3
    shift-left: w9 -> [w141]
    stop <- w142 continue-if-true
    # "continue while falling bricks detected"
    n76 = call "Detect unsuported Brick and fall.vi"("Grid"=w141, "Brick Map"=w145) -> ("Continue"=w142:bool, "Grid out"=w143:i32[][][], "Brick Map"=w144:map{i32, T1[]})  [unwired: 7 in]
  }
  "Grid" <- w3
  "Brick Map" <- w2
  n77 = call "Scan Page find supports.vi"("Block Array"=w3) -> ("Support Map"=w7:map{i32, set{i32}})  [unwired: 10 in]
  n78 = call "Find keeper counts.vi"("Support Map"=w7, "Brick Map"=w2) -> ("Keep Map"=w6:map{i32, T2})  [unwired: 9 in]
  n79 = for {
    tunnel: w6 -> [w151] mode=indexing
    tunnel: w6 -> [w152]
    tunnel: [w148] -> w5 mode=indexing
    tunnel: w3 -> [w147]
    tunnel: w2 -> [w146]
    n80 = Unbundle By Name(w151) -> ("Dependancies.keep"=w150:bool, "ID"=w149:i32)
    n81 = case shown="True" w150 {
      tunnel: w152 -> [_ w162]
      tunnel: w149 -> [_ w157]
      tunnel: [0 ("size") w159] -> w148
      tunnel: w147 -> [_ w155]
      tunnel: w146 -> [_ w158]
      frame False {
      }
      frame True {
        n82 = Look In Map(map=w158, key=w157) -> (value=w156:T1[])  [unwired: 1 in, 1 out]
        n83 = for {
          tunnel: w156 -> [w169] mode=indexing
          shift-right: [w167] -> w154
          shift-left: w155 -> [w168]
          n84 = Unbundle By Name(w169) -> ("Page"=w166:i32, "Row"=w165:i32, "Col"=w164:i32)
          n85 = Replace Array Subset(array=w168, new element=0, index (dim 0)=w166, index (dim 1)=w165, index (dim 2)=w164) -> (w167:i32[][][])
        }
        n86 = while {
          tunnel: w162 -> [_]
          shift-right: [w175] -> w160
          shift-left: set{i32} {} ("Dropped Set") -> [w176]
          shift-right: [w172] -> _
          shift-left: w154 -> [w170]
          shift-right: [w173] -> _
          shift-left: w158 -> [w171]
          stop <- w174 continue-if-true
          n87 = call "Detect unsuported Brick and fall and keep track.vi"("Dropped Set"=w176, "Grid"=w170, "Brick Map"=w171) -> ("Continue"=w174:bool, "Grid out"=w172:i32[][][], "Brick Map"=w173:map{i32, T1[]}, "Dropped Set"=w175:set{i32})  [unwired: 5 in]
        }
        n88 = Collection Size(1:w160) -> (0:w159:i32)
      }
    }
  }
  n89 = Add Array Elements(numeric array=w5) -> (sum=→"Answer":i32)
